vi "Refresh SRs.vi"(8 "error in":errorcluster, 11 "Data Loop Data in":T1) -> (0 "error out":errorcluster, 3 "Data Loop Data out":T1)   [LabVIEW 2018]
uses:
  Type Defs/Data Loop Data.ctl
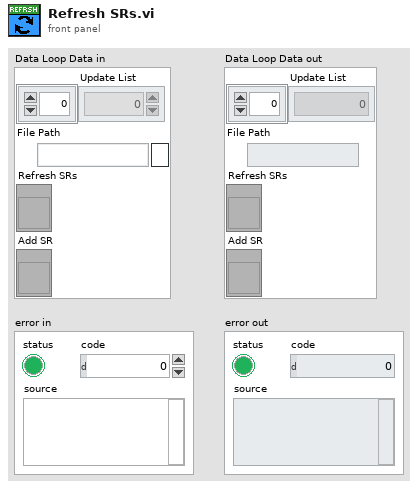
[diagram p1: front panel]
types:
  T1 = typedef "Data Loop Data.ctl" = cluster{"Update List":i32[], "File Path":path, "Refresh SRs":refnum<vi>, "Add SR":refnum<vi>}
  T2 = typedef "SR Cluster.ctl" = cluster{"Color":u32, "SR Number":i32, "SR Status":T3, "Name":string, "Summary":string, "Last Updated":timestamp, "SR Type":string, "Service Level":string, "Days Open":dbl, "Creation Date":timestamp}
  T3 = typedef "SR Status.ctl" = enum16{"Caller Abandoned", "Created in Error", "Expired", "Forum Resolved AE", "Forum Resolved Customer", "IN WORK", "IN WORK Collab with AES", "IN WORK Collab with PSE", "IN WORK Collab with SE", "IN WORK Customer Added Note", "IN WORK Escalation", "IN WORK Wait on Customer", "Open", "Potentially Resolved", "Presumed Resolved", "RMA Approved for Return", "Resolved", "Passed Off"}
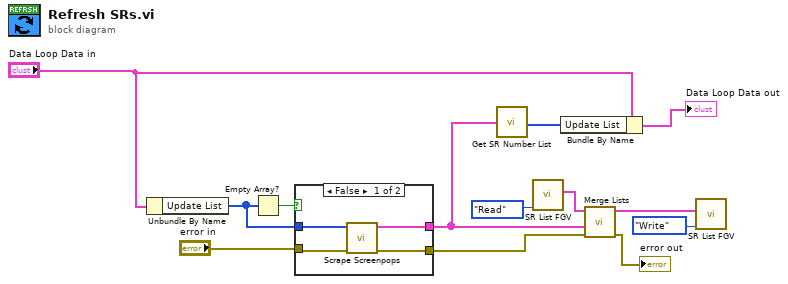
[diagram p0: block diagram]
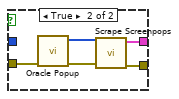
[diagram p2: hidden frame]
diagram:
  n1 = Unbundle By Name("Data Loop Data in") -> ("Update List"=w4:i32[])
  n2 = Empty Array?(array=w4) -> (empty?=w5:bool)
  n3 = case shown="False" w5 {
    tunnel: [w15 w22] -> w10
    tunnel: [w16 w21] -> w1
    tunnel: w4 -> [w17 _]
    tunnel: "error in" -> [w14 w18]
    frame False {
      n4 = call "Scrape Screenpops.vi"("error in"=w14, "SR number list in"=w17) -> ("error out"=w15:errorcluster, "sr clusters out"=w16:T2[])  [unwired: 8 in]
    }
    frame True {
      n5 = call "Oracle Popup.vi"("error in"=w18) -> ("error out"=w19:errorcluster, "SR array out"=w20:i32[])  [unwired: 9 in]
      n6 = call "Scrape Screenpops.vi"("error in"=w19, "SR number list in"=w20) -> ("error out"=w22:errorcluster, "sr clusters out"=w21:T2[])  [unwired: 8 in]
    }
  }
  n7 = call "Get SR Number List.vi"("list in"=w1) -> ("SR number array out"=w2:i32[])  [unwired: 4 in]
  n8 = call "SR List FGV.vi"("Operation"=enum16{"Initialize", "Write", "Read", "Clear"}."Read") -> ("list out"=w13:T2[])  [unwired: 9 in, 1 out]
  n9 = Bundle By Name(cluster="Data Loop Data in", "Update List"=w2) -> (→"Data Loop Data out":T1)
  n10 = call "Merge Lists.vi"("error in"=w10, "new list in"=w1, "list in"=w13) -> ("error out"=→"error out":errorcluster, "list out"=w12:T2[])  [unwired: 7 in]
  n11 = call "SR List FGV.vi"("Operation"=enum16{"Initialize", "Write", "Read", "Clear"}."Write", "list in"=w12) -> ()  [unwired: 8 in, 2 out]
